vi "Stop Core.vi"(10 "final error code":i32, 11 "Nested in":refnum<class "C100L.lvclass">) -> (3 "Nested out":refnum<class "C100L.lvclass">)   [LabVIEW 2021, in "C100L.lvlib" / "C100L.lvclass"]
doc: "(<B>Filename</B>: Actor Framework.lvlib:Actor.lvclass:Stop Core.vi)\n\nDefines what the actor does before it stops. Use the <B>final error code</B> input to determine whether the actor shut down in response to an error.\n\nBy default, this method does nothing. A descendant class may override it to define behavior, such as shutting down any processes the actor initiated in its override of the Actor Core method."
uses:
  C100L.lvclass
  <vilib>/MGI/Panel Manager/Panel Actor/Panel Actor/Panel Actor.lvclass
  C100L.lvclass/C100L.ctl
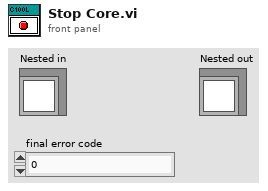
[diagram p1: front panel]
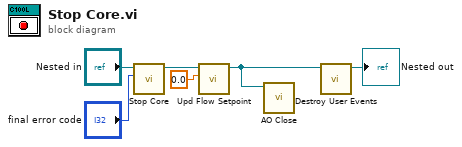
[diagram p0: block diagram]
diagram:
  n1 = call-parent "Stop Core.vi"("final error code"="final error code", "Actor in"="Nested in") -> ("Actor out"=w3:refnum<class "C100L.lvclass">)  [unwired: 9 in]
  n2 = call "Upd Flow Setpoint.vi"("Flow Setpoint"=0.0, "C100L in"=w3) -> ("C100L out"=w1:refnum<class "C100L.lvclass">)  [unwired: 8 in, 1 out]
  n3 = call "AO Close.vi"("C100L in"=w1) -> ()  [unwired: 10 in, 1 out]
  n4 = call "Destroy User Events.vi"("UI Template in"=w1) -> ("UI Template out"=→"Nested out":refnum<class "C100L.lvclass">)  [unwired: 10 in]
